vi "Method 3 Ultrasonic.vi"   [LabVIEW 2012]
uses:
  <vilib>/NXT/Subs/MotorOutput.ctl
  <vilib>/NXT/Block Support/NXT_InputPort.ctl
types:
  T1 = typedef "MotorOutput.ctl" = u8
  T2 = typedef "NXT_InputPort.ctl" = u32
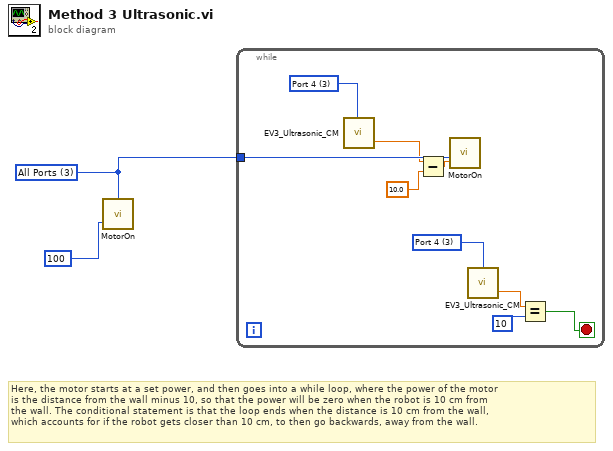
[diagram p0: block diagram]
diagram:
  w1 = T1 3 items=["Port A"=0, "Port B"=1, "Port C"=2, "Ports A & B"=4, "Ports A & C"=5, "Ports B & C"=6, "All Ports"=3] ("Output Port (All Ports)")
  # "Here, the motor starts at a set power, and then goes into a while loop, where the power of the motor\nis the distance from the wall minus 10, so that the power will be zero when the robot is 10 cm from \nthe wall. The conditional statement is that the loop ends when the distance is 10 cm from the wall, \nwhich accounts for if the robot gets closer than 10 cm, to then go backwards, away from the wall."
  n1 = call <vilib>:"MotorOn.vi"("Power (75)"=100, "Output Port (All Ports)"=w1) -> ()  [unwired: 2 in, 1 out]
  n2 = while {
    tunnel: w1 -> [w11]
    stop <- w3 stop-if-true
    w4 = T2 3 items=["Port 1", "Port 2", "Port 3", "Port 4"] ("Port (Port 1)")
    w7 = T1 3 items=["Port A"=0, "Port B"=1, "Port C"=2, "Ports A & B"=4, "Ports A & C"=5, "Ports B & C"=6, "Port 4"=3] ("Output Port (All Ports)")
    n3 = call <vilib>:"EV3_Ultrasonic_CM.vi"("Port (Port 1)"=w7) -> ("Centimeters"=w10:sgl)  [unwired: 2 in, 1 out]
    n4 = Subtract(x=w10, y=sgl 10.0) -> (x-y=w8:sgl)
    n5 = call <vilib>:"MotorOn.vi"("Power (75)"=w8, "Output Port (All Ports)"=w11) -> ()  [unwired: 2 in, 1 out]
    n6 = call <vilib>:"EV3_Ultrasonic_CM.vi"("Port (Port 1)"=w4) -> ("Centimeters"=w5:sgl)  [unwired: 2 in, 1 out]
    n7 = Equal?(x=w5, y=10) -> (x = y?=w3:bool)
  }
